vi "Read Analogue.vi"(8 "error in (no error)":errorcluster, 11 "NI Scope":refnum<class "NI Scope.lvclass">) -> (0 "error out":errorcluster, 2 "Waveforms":waveform(dbl)[](array[waveform]), 3 "NI Scope out":refnum<class "NI Scope.lvclass">)   [LabVIEW 2025, in "Scope.lvlib" / "NI Scope.lvclass"]
uses:
  NI Scope.lvclass
  NI Scope.lvclass/NI Scope.ctl
  <instrlib>/niScope/Acquire/niScope Multi Read WDT.vi
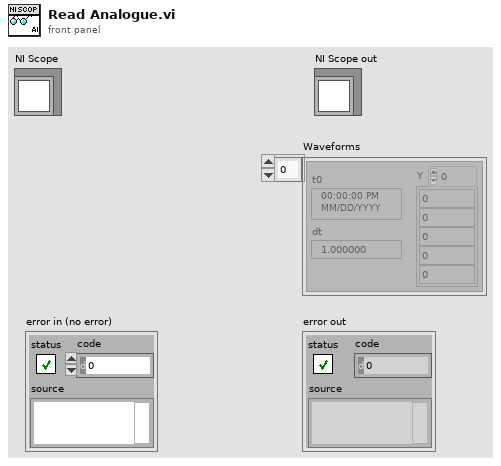
[diagram p1: front panel]
types:
  T1 = typedef "Abstract Engine.lvlibp/Abstract Instrument.lvclass/Channel.ctl" = cluster{"Alias":string, "DataType":enum16{"Anaolg Input", "Waveform"}, "Unit":enum16{"---", "V", "A", "Ohm", "Hz", "uF", "degC", "deg"}, "Upper limit":dbl, "Lower limit":dbl, "Measurement":variant}
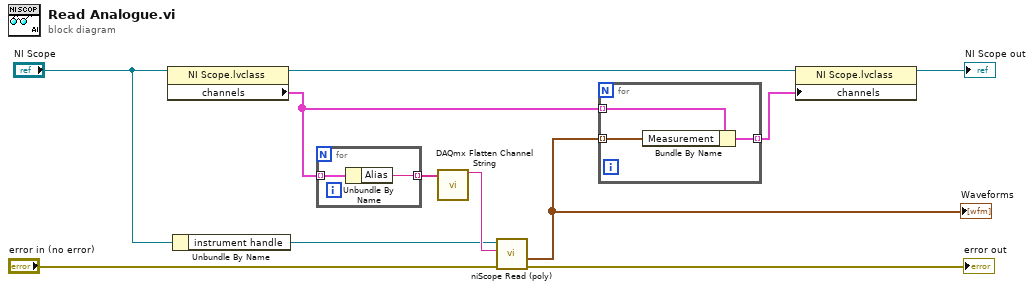
[diagram p0: block diagram]
diagram:
  n1 = property class="NI Scope.lvclass"(reference="NI Scope") -> (reference out=w8:refnum<class "NI Scope.lvclass">, "channels"=w9:T1[])  [unwired: 1 in, 1 out]
  n2 = Unbundle By Name("NI Scope") -> ("instrument handle"=w7:refnum<k15>)
  n3 = for {
    tunnel: w9 -> [w13] mode=indexing
    tunnel: [w12] -> w10 mode=indexing
    n4 = Unbundle By Name(w13) -> ("Alias"=w12:string)
  }
  n5 = call <vilib>:"DAQmx Flatten Channel String.vi"("names in"=w10) -> ("names out"=w11:string)  [unwired: 13 in, 1 out]
  n6 = call-poly <instrlib>:"niScope Read (poly).vi"("error in"="error in (no error)", "channels"=w11, "instrument handle"=w7) -> ("error out"=→"error out":errorcluster, "wfm"=w1:waveform(dbl)[])  [unwired: 5 in, 2 out]
  "Waveforms" <- w1
  n7 = for {
    tunnel: w1 -> [w16] mode=indexing
    tunnel: w9 -> [w14] mode=indexing
    tunnel: [w15] -> w2 mode=indexing
    n8 = Bundle By Name(cluster=w14, "Measurement"=w16) -> (w15:T1)
  }
  n9 = property class="NI Scope.lvclass"(reference=w8, "channels"=w2) -> (reference out=→"NI Scope out":refnum<class "NI Scope.lvclass">)  [unwired: 1 in, 1 out]
